vi "Lee_csv.vi"(0 "Path":path) -> (1 "Tabla_flota":string[][](array[string]), 2 "Lectura_OK?":bool)   [LabVIEW 2015]
uses:
  <vilib>/Utility/file.llb/Read Delimited Spreadsheet (string).vi
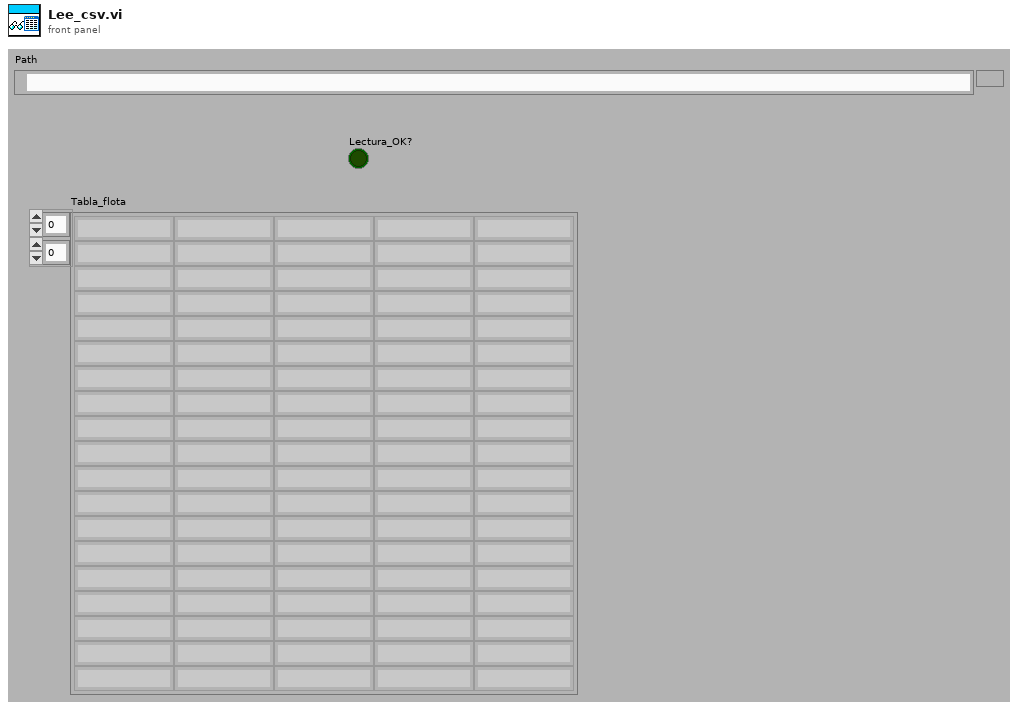
[diagram p1: front panel]
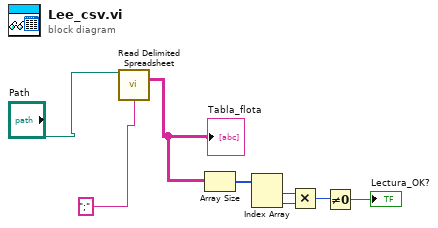
[diagram p0: block diagram]
diagram:
  n1 = call-poly <vilib>:"Read Delimited Spreadsheet.vi"("file path (dialog if empty)"="Path", "delimiter (\\t)"=";" ("delimiter (\\t)")) -> ("all rows"=w2:string[][])  [unwired: 8 in, 5 out]
  "Tabla_flota" <- w2
  n2 = Array Size(array=w2) -> (size(s)=w8:i32[])
  n3 = Index Array(array=w8) -> (element #1=w6:i32, element #2=w7:i32)  [unwired: 2 in]
  n4 = Multiply(x=w6, y=w7) -> (x*y=w5:i32)
  n5 = Not Equal To 0?(x=w5) -> (x != 0?=→"Lectura_OK?":bool)
